vi "Configure Valve Opening Offset.vi"(8 "error in (no error)":errorcluster, 9 "offset":sgl, 10 "node address (same)":u8, 11 "ProPar in":refnum<class "PL Bronkhorst ProPar.lvclass">) -> (0 "error out":errorcluster, 3 "ProPar out":refnum<class "PL Bronkhorst ProPar.lvclass">)   [LabVIEW 2015, in "PL Bronkhorst ProPar.lvclass"]
doc: "Configures first-step offset current/voltage for valve when opening from 0% of the specified <b>node</b>."
uses:
  PL Bronkhorst ProPar.lvclass
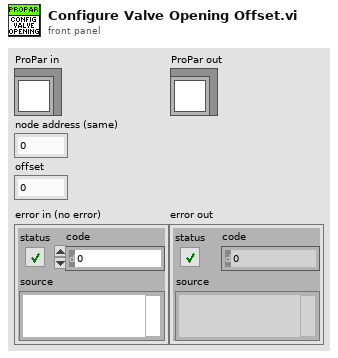
[diagram p1: front panel]
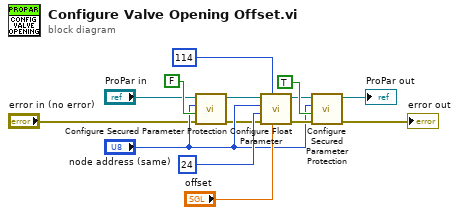
[diagram p0: block diagram]
diagram:
  n1 = call "Configure Secured Parameter Protection.vi"("error in (no error)"="error in (no error)", "enable protection"=FALSE, "node"="node address (same)", "ProPar in"="ProPar in") -> ("error out"=w3:errorcluster, "ProPar out"=w2:refnum<class "PL Bronkhorst ProPar.lvclass">)  [unwired: 6 in]
  n2 = call "Configure Float Parameter.vi"("value"="offset", "process number"=u8 114, "error in (no error)"=w3, "parameter number"=u8 24 ("process number"), "node"="node address (same)", "ProPar in"=w2) -> ("error out"=w8:errorcluster, "ProPar out"=w6:refnum<class "PL Bronkhorst ProPar.lvclass">)  [unwired: 4 in]
  n3 = call "Configure Secured Parameter Protection.vi"("error in (no error)"=w8, "enable protection"=TRUE, "node"="node address (same)", "ProPar in"=w6) -> ("error out"=→"error out":errorcluster, "ProPar out"=→"ProPar out":refnum<class "PL Bronkhorst ProPar.lvclass">)  [unwired: 6 in]
